vi "DistanceSensor SonarReflections Example.vi"() -> ()   [LabVIEW 2012, in "Phidget Distance Sensor.lvlib"]
uses:
  <instrlib>/Phidgets/Phidget Distance Sensor/Phidget Distance Sensor.lvlib
  <instrlib>/Phidgets/Phidget Distance Sensor/Public/DistanceSensorStart.vi
  <instrlib>/Phidgets/Phidget Distance Sensor/Public/DistanceSensorClose.vi
  <instrlib>/Phidgets/Phidget Common/Phidget Common.lvlib
panel:
  out "Count":u32
  out "Amplitudes":u32[](array[numeric])
  out "Distances":u32[](array[numeric])
  out "error out":errorcluster
  in  "error in (no error)":errorcluster
  in  "Device Info":T1={"Serial Number"=-1, "Channel"=0, "Port"=0}
  out "Attached?":bool
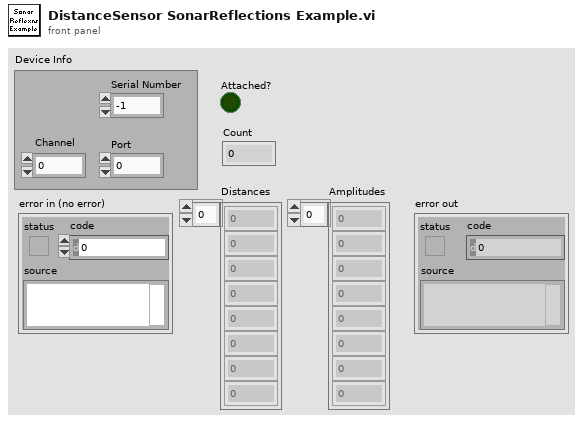
[diagram p1: front panel]
types:
  T1 = cluster{"Serial Number":i32, "Channel":i32, "Port":i32}
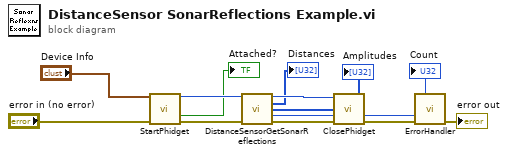
[diagram p0: block diagram]
diagram:
  n1 = call-poly <instrlib>:"StartPhidget.vi"("Device Info"="Device Info", "error in (no error)"="error in (no error)") -> ("Phidget ID"=w12:u64, "Attached?"=→"Attached?":bool, "error out"=w11:errorcluster)  [unwired: 10 in, 1 out]
  n2 = call <instrlib>:"DistanceSensorGetSonarReflections.vi"("Device In"=w12, "error in (no error)"=w11) -> ("Device Out"=w5:u64, "Distances"=→"Distances":u32[], "Amplitudes"=→"Amplitudes":u32[], "Count"=→"Count":u32, "error out"=w4:errorcluster)  [unwired: 9 in]
  n3 = call-poly <instrlib>:"ClosePhidget.vi"("error in"=w4, "Device In"=w5) -> ("error out"=w7:errorcluster)  [unwired: 9 in]
  n4 = call <instrlib>:"ErrorHandler.vi"("error in"=w7) -> ("error out"=→"error out":errorcluster)  [unwired: 9 in, 1 out]
